vi "LVClass_HasoEngine dtor.vi"(0 "HasoEngine in":refnum<class "HasoEngine.lvclass">, 11 "error in (no error)":errorcluster) -> (4 "HasoEngine out":refnum<class "HasoEngine.lvclass">, 15 "error out":errorcluster)   [LabVIEW 2020, in "HasoEngine.lvclass"]
doc: "HasoEngine destructor.\n\n--------------------------------------------------------------------------------\n\n<B>HasoEngineIn </B> : HasoEngine object.\n<B>HasoEngineOut </B> : HasoEngine object.\n<B>ErrorIn </B> : Error\n<B>ErrorOut </B> : Error\n\n--------------------------------------------------------------------------------"
uses:
  HasoEngine.lvclass
  HasoEngine.lvclass/HasoEngine.ctl
  HasoSlopes/HasoSlopes.lvclass
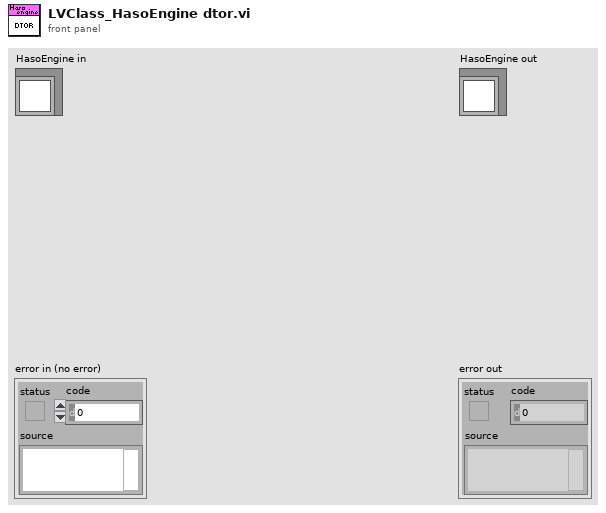
[diagram p1: front panel]
types:
  T1 = typedef "Handle creation.ctl" = enum16{"By ctor", "By write function"}
  T2 = typedef "ClassID.ctl" = i64
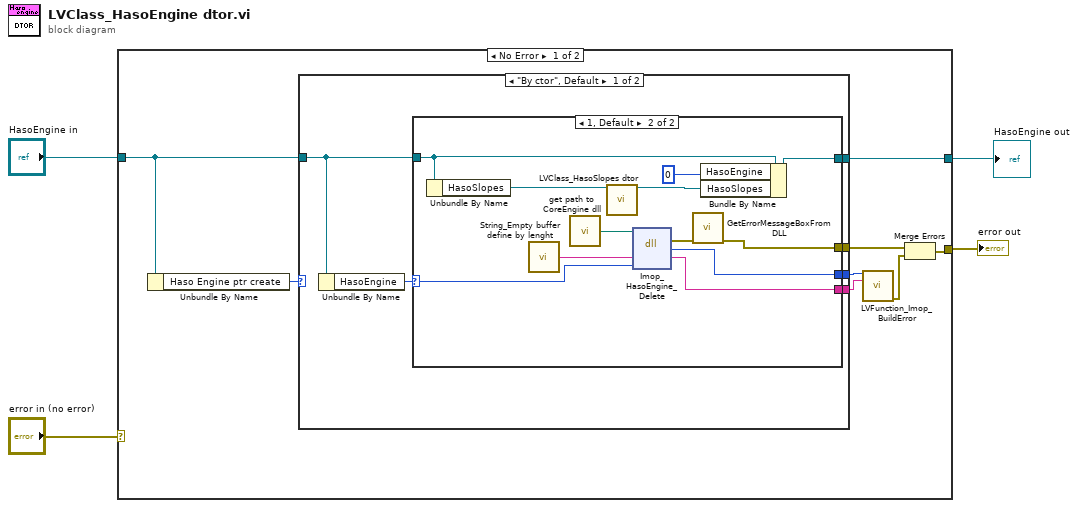
[diagram p0: block diagram]
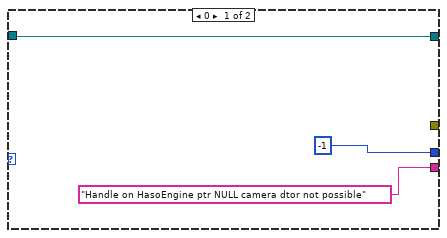
[diagram p2: hidden frame]
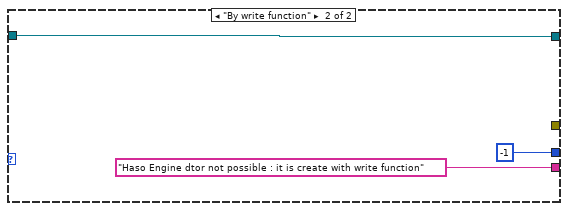
[diagram p3: hidden frame]
diagram:
  n1 = case shown="No Error" "error in (no error)" {
    selector: "error in (no error)" -> [_ w37]
    tunnel: "HasoEngine in" -> [w9 w38]
    tunnel: [w10 w38] -> w1
    tunnel: [w5 w37] -> w2
    frame No Error {
      n2 = Unbundle By Name(w9) -> ("Haso Engine ptr create"=w8:T1)
      n3 = case shown="\"By ctor\", Default" w8 {
        tunnel: [w18 "Haso Engine dtor not possible : it is create with write function" ("message")] -> w12
        tunnel: [w17 -1] -> w11
        tunnel: w9 -> [w15 w34]
        tunnel: [w16 w34] -> w10
        tunnel: [w13 _] -> w7
        frame "By ctor", Default {
          n4 = Unbundle By Name(w15) -> ("HasoEngine"=w14:T2)
          n5 = case shown="1, Default" w14 {
            selector: w14 -> [_ w30]
            tunnel: ["Handle on HasoEngine ptr NULL camera dtor not possible" ("message") w32] -> w18
            tunnel: [-1 w31] -> w17
            tunnel: w15 -> [w19 w25]
            tunnel: [w19 w26] -> w16
            tunnel: [_ w23] -> w13
            frame 0 {
            }
            frame 1, Default {
              n6 = Unbundle By Name(w25) -> ("HasoSlopes"=w24:refnum<class "HasoSlopes.lvclass">)
              n7 = call "String_Empty buffer define by lenght.vi"() -> ("Empty buffer"=w33:string)  [unwired: 1 in]
              n8 = call "get path to CoreEngine dll.vi"() -> ("path to wavekit library"=w29:path)  [unwired: 14 in, 1 out]
              n9 = call "LVClass_HasoSlopes dtor.vi"("HasoSlopes in"=w24) -> ("HasoSlopes out"=w22:refnum<class "HasoSlopes.lvclass">)  [unwired: 13 in, 1 out]
              n10 = dll-call lib="D:/soft/HASO_v3/SVN_trunk/ImOpCoreEngine4_LV2011/DLLs/c_interface_vc100.dll" fn="Imop_HasoEngine_Delete"(path in=w29, "message"=w33, "objet"=w30) -> (error out=w28:errorcluster, "return type"=w31:i32, "message"=w32:string)  [unwired: 3 in, 1 out]
              n11 = call "GetErrorMessageBoxFromDLL.vi"("error IN"=w28) -> ("error OUT"=w23:errorcluster)  [unwired: 10 in]
              n12 = Bundle By Name(cluster=w25, "HasoEngine"=u32 0 ("HasoEgine"), "HasoSlopes"=w22) -> (w26:refnum<class "HasoEngine.lvclass">)
            }
          }
        }
        frame "By write function" {
        }
      }
      n13 = call "LVFunction_Imop_BuildError.vi"("code"=w11, "String to Prepend to source (\"\")"=w12) -> ("error out"=w6:errorcluster)  [unwired: 13 in]
      n14 = Merge Errors(w7, w6) -> (w5:errorcluster)
    }
    frame Error {
    }
  }
  "error out" <- w2
  "HasoEngine out" <- w1
